vi "System_Conf_RW.vi"(7 "Mode":enum16{"Read", "Write"}(ring), 8 "error in":errorcluster, 11 "system":T1={"空载滤波"=FALSE, "逆向空载滤波"=FALSE, "空载扭矩系数"=1.0, "逆向空载扭矩系数"=1.0}) -> (0 "error out":errorcluster, 3 "system_out":T1)   [LabVIEW 2020]
uses:
  From/System_conf.ctl
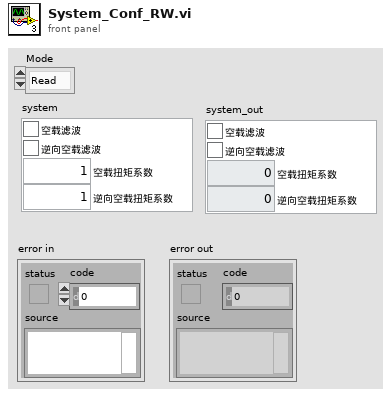
[diagram p1: front panel]
types:
  T1 = typedef "System_conf.ctl" = cluster{"空载滤波":bool, "逆向空载滤波":bool, "空载扭矩系数":dbl, "逆向空载扭矩系数":dbl}
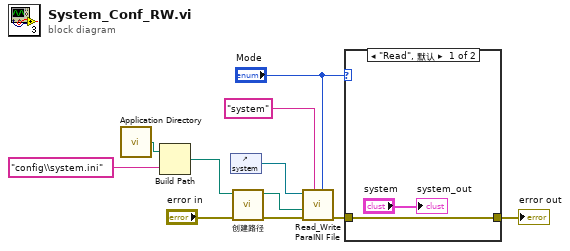
[diagram p0: block diagram]
diagram:
  n1 = call <vilib>:"Application Directory.vi"() -> ("Application Directory"=w10:path)
  n2 = Build Path(base path=w10, name or relative path="config\\system.ini" ("名称或相对路径")) -> (appended path=w4:path)
  n3 = control-ref of="system"() -> (w11:refnum<vi>)
  n4 = call "创建路径.vi"("error in (no error)"="error in", "path"=w4) -> ("error out"=w1:errorcluster, "path out"=w3:path)  [unwired: 8 in]
  n5 = call "Read_Write ParaINI File.vi"("Mode"="Mode", "Section"="system", "error in"=w1, "Filepath"=w3, "Ctl Refnum"=w11) -> ("error out"=w6:errorcluster)  [unwired: 6 in]
  n6 = case shown="\"Read\", 默认" "Mode" {
    tunnel: w6 -> [w12 w14]
    tunnel: [w12 w14] -> w5
    frame "Read", Default {
      "system_out" <- "system"
    }
    frame "Write" {
    }
  }
  "error out" <- w5
